vi "Axsun VDL Global.vi"() -> ()   [LabVIEW 2015, in "Axsun_1310_SS.lvclass"]
uses:
  Axsun_1310_SS.lvclass
  C:/Program Files (x86)/Axsun/Axsun OCT Control/AxsunOCTControl.dll
  Axsun VDL Typedef.ctl
panel:
  in  "VDL Inputs":T1 {"Position (mm)" min=0.0 max=15.0 scale=0.0..15.0; "Speed (mm/s)" min=0.0 max=7.0 scale=0.0..7.0}
  in  "Axsun .NET Ref":refnum<k24>
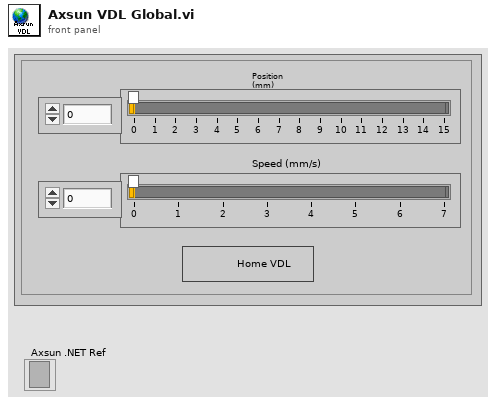
[diagram p1: front panel]
types:
  T1 = typedef "Axsun_1310_SS.lvclass/Axsun VDL Typedef.ctl" = cluster{"Speed (mm/s)":dbl, "Position (mm)":dbl, "Home":bool}
diagram:
